vi "Serialize as VTT.vi"(8 "error in (no error)":errorcluster, 11 "Reference in":refnum<class "Reference.lvclass">) -> (0 "error out":errorcluster, 2 "VTT Fragment":string, 3 "Reference out":refnum<class "Reference.lvclass">)   [LabVIEW 2020, in "VILab.lvlib" / "Reference.lvclass"]
uses:
  Reference.lvclass
  C:/Users/User/Documents/LabVIEW Data/Projects/VILab/source/SubVIs/Classes/Element/Element.lvclass
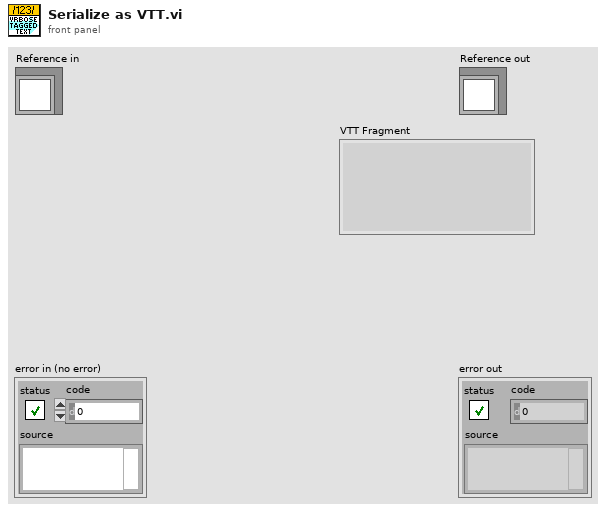
[diagram p1: front panel]
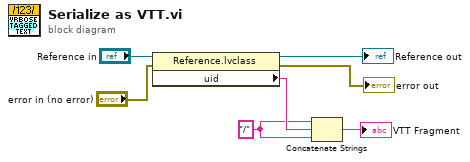
[diagram p0: block diagram]
diagram:
  w1 = "/"
  n1 = property class="Reference.lvclass"(reference="Reference in", error in="error in (no error)") -> (reference out=→"Reference out":refnum<class "Reference.lvclass">, error out=→"error out":errorcluster, "uid"=w2:string)
  n2 = Concatenate Strings(w1, w2, w1) -> (→"VTT Fragment":string)
